vi "CAN Jaguar Config Brake Coast.vi"(8 "error in (no error)":errorcluster, 10 "Brake / Coast Mode":T1, 11 "CAN Jaguar Ref":T2={"Device Number"=0, "Control Mode"=enum."Percent VBus", "Inverted"=FALSE, "Semaphore"=refnum, "Max Vout"=12.0, "DevStatus"={"status"=FALSE, "code"=0, "source"=""}}) -> (0 "error out":errorcluster, 3 "CAN Jaguar Ref Out":T2={"Device Number"=0, "Control Mode"=enum."Percent VBus", "Inverted"=FALSE, "Semaphore"=refnum, "Max Vout"=12.0, "DevStatus"={"status"=FALSE, "code"=0, "source"=""}})   [LabVIEW 2009, in "CAN.lvlib"]
uses:
  CAN.lvlib
  SubVIs/CAN Jaguar Ref.ctl
  SubVIs/CAN Jaguar Control Mode.ctl
  SubVIs/CAN Jaguar Brake Coast Mode.ctl
  SubVIs/CAN Motor Message IDs.ctl
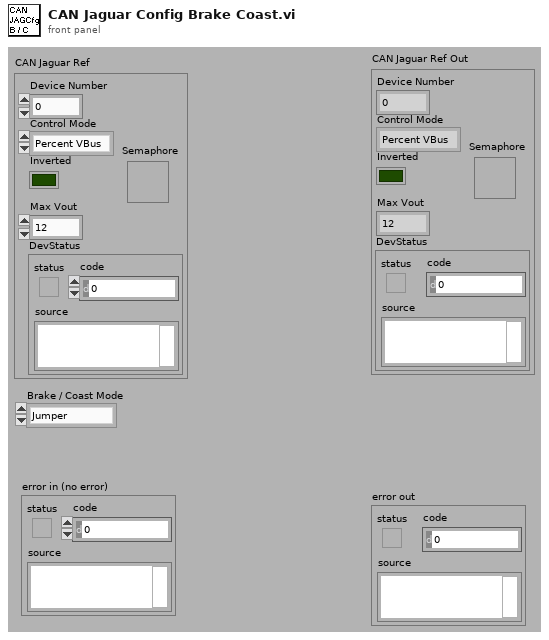
[diagram p1: front panel]
types:
  T1 = typedef "CAN.lvlib/CAN Jaguar Brake Coast Mode.ctl" = enum16{"Jumper", "Brake", "Coast"}
  T2 = typedef "CAN.lvlib/CAN Jaguar Ref.ctl" = cluster{"Device Number":u8, "Control Mode":T3, "Inverted":bool, "Semaphore":T4, "Max Vout":dbl, "DevStatus":errorcluster}
  T3 = typedef "CAN.lvlib/CAN Jaguar Control Mode.ctl" = enum16{"Percent VBus", "Speed", "Position", "Current"}
  T4 = typedef "Semaphore RefNum" = refnum<k1>
  T5 = enum16{"big-endian, network order", "native, host order", "little-endian"}
  T6 = typedef "CAN.lvlib/CAN Motor Message IDs.ctl" = u32
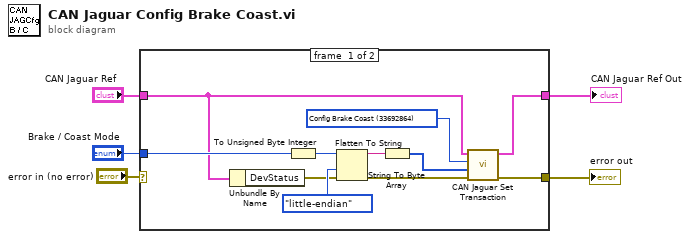
[diagram p0: block diagram]
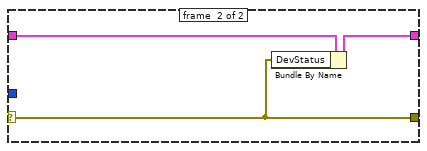
[diagram p2: hidden frame]
diagram:
  n1 = case shown="No Error" "error in (no error)" {
    selector: "error in (no error)" -> [_ w17]
    tunnel: [w10 w17] -> w5
    tunnel: [w8 w18] -> w3
    tunnel: "CAN Jaguar Ref" -> [w9 w19]
    tunnel: "Brake / Coast Mode" -> [w16 _]
    frame #0 {
      w6 = T6 33692864 items=["Volt Enable"=33685504, "Volt Disable"=33685568, "Volt Set"=33685632, "Volt Set Ramp"=33685696, "Speed Enable"=33686528, "Speed Disable"=33686592, "Speed Set"=33686656, "Speed P"=33686720, "Speed I"=33686784, "Speed D"=33686848, "Speed Ref"=33686912, "Position Enable"=33688576, "Position Disable"=33688640, "Position Set"=33688704, "Position P"=33688768, "Position I"=33688832, "Position D"=33688896, "Position Ref"=33688960, "Current Enable"=33689600, "Current Disable"=33689664, "Current Set"=33689728, "Current P"=33689792, "Current I"=33689856, "Current D"=33689920, "Status VOut"=33690624, "Status VBus"=33690688, "Status Current"=33690752, "Status Temp"=33690816, "Status Position"=33690880, "Status Speed"=33690944, "Status Limit"=33691008, "Status Fault"=33691072, "Status Power"=33691136, "Config Num Brushes"=33692672, "Config Encoder Lines"=33692736, "Config Pot Turns"=33692800, "Config Brake Coast"=33692864, "Config Limit Mode"=33692928, "Config Limit Fwd"=33692992, "Config Limit Rev"=33693056, "Config Max VOut"=33693120, "Config Fault Time"=33693184, "Motor Ack"=33693696] ("CAN Motor Message IDs")
      n2 = Unbundle By Name(w9) -> ("DevStatus"=w12:errorcluster)
      n3 = To Unsigned Byte Integer(number=w16) -> (unsigned 8bit integer=w13:u8)
      n4 = Flatten To String(anything=w13, byte order (0:big-endian, network order)=T5."little-endian", error in (no error)=w12) -> (data string=w14:string, error out=w11:errorcluster)  [unwired: 2 out]
      n5 = String To Byte Array(string=w14) -> (unsigned byte array=w7:u8[])
      n6 = call "CAN Jaguar Set Transaction.vi"("error in"=w11, "Data"=w7, "Message ID"=w6, "CAN Jaguar Ref"=w9) -> ("error out"=w10:errorcluster, "CAN Jaguar Ref Out"=w8:T2)  [unwired: 6 out]
    }
    frame #1 {
      n7 = Bundle By Name(cluster=w19, "DevStatus"=w17) -> (w18:T2)
    }
  }
  "CAN Jaguar Ref Out" <- w3
  "error out" <- w5
